vi "practica111.vi"() -> ()   [LabVIEW 2016]
panel:
  out "S2 x":dbl
  out "S2 y":dbl
  out "S1 x":dbl
  out "S1 y":dbl
  in  "S2":i32
  in  "S1":i32
  in  "stop":bool
  in  "S2":dbl(knob) scale=-175.0..175.0
  in  "S1":dbl(knob) scale=0.0..360.0
  out "XY Graph":cluster{"Y":dbl[], "Y":dbl[]}[](graph)
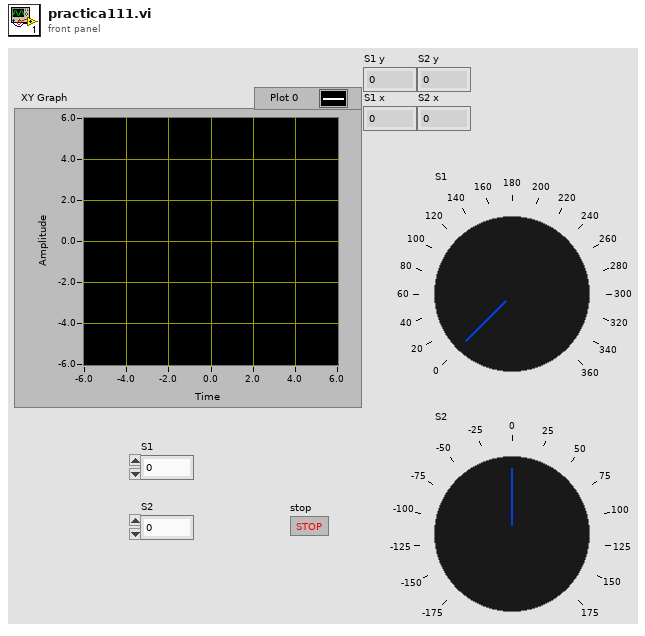
[diagram p1: front panel]
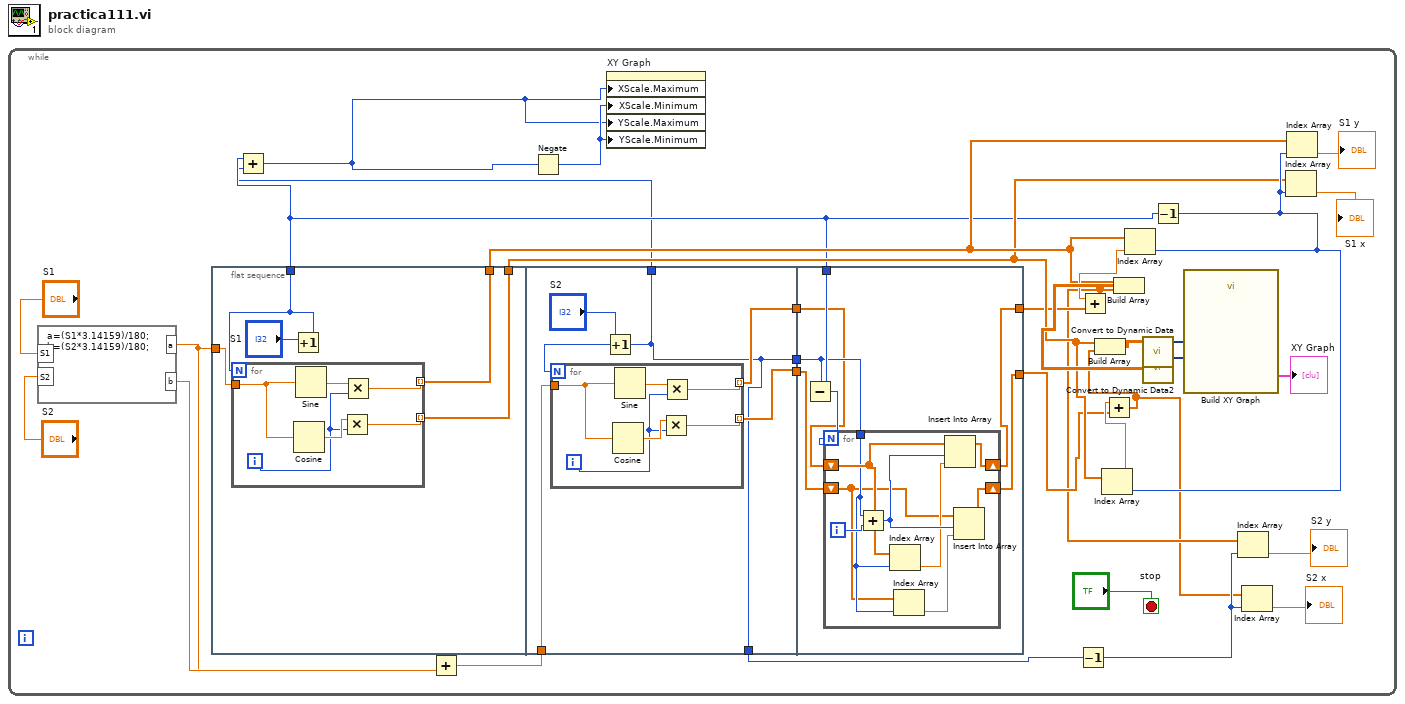
[diagram p0: block diagram]
diagram:
  n1 = while {
    stop <- "stop" stop-if-true
    n2 = formula code="a=(S1*3.14159)/180;\nb=(S2*3.14159)/180;"("S1"="S1", "S2"="S2") -> ("b"=w24:dbl, "a"=w23:dbl)
    n3 = flat-sequence {
      tunnel: w23 -> [w38]
      tunnel: [w34] -> w4
      tunnel: [w36] -> w16
      tunnel: [w35] -> w15
      tunnel: w22 -> [w48]
      tunnel: [w47] -> w20
      tunnel: [w46] -> w19
      tunnel: [w45] -> w18
      tunnel: [w45] -> w7
      tunnel: [w45] -> w3
      tunnel: [w59] -> w12
      tunnel: [w58] -> w9
      tunnel: w20 -> [w56]
      tunnel: w19 -> [w57]
      tunnel: w4 -> [w62]
      tunnel: w18 -> [w60]
      frame #0 {
        n4 = Increment(x="S1") -> (x+1=w34:i32)
        n5 = for {
          N: w34 -> [_]
          tunnel: w38 -> [w40]
          tunnel: [w42] -> w36 mode=indexing
          tunnel: [w41] -> w35 mode=indexing
          i -> [w39]
          n6 = Cosine(x=w40) -> (cos(x)=w44:dbl)
          n7 = Sine(x=w40) -> (sin(x)=w43:dbl)
          n8 = Multiply(x=w44, y=w39) -> (x*y=w41:dbl)
          n9 = Multiply(x=w43, y=w39) -> (x*y=w42:dbl)
        }
      }
      frame #1 {
        n10 = Increment(x="S2") -> (x+1=w45:i32)
        n11 = for {
          N: w45 -> [_]
          tunnel: w48 -> [w51]
          tunnel: [w53] -> w46 mode=indexing
          tunnel: [w52] -> w47 mode=indexing
          i -> [w50]
          n12 = Cosine(x=w51) -> (cos(x)=w55:dbl)
          n13 = Sine(x=w51) -> (sin(x)=w54:dbl)
          n14 = Multiply(x=w55, y=w50) -> (x*y=w52:dbl)
          n15 = Multiply(x=w54, y=w50) -> (x*y=w53:dbl)
        }
      }
      frame #2 {
        n16 = Subtract(x=w62, y=w60) -> (x-y=w61:i32)
        n17 = for {
          N: w61 -> [_]
          tunnel: w60 -> [w66]
          shift-right: [w67] -> w59
          shift-left: w57 -> [w69]
          shift-right: [w63] -> w58
          shift-left: w56 -> [w65]
          i -> [w71]
          n18 = Add(x=w66, y=w71) -> (x+y=w70:i32)
          n19 = Index Array(array=w69, index=w66) -> (element=w68:dbl)
          n20 = Index Array(array=w65, index=w66) -> (element=w64:dbl)
          n21 = Insert Into Array(array=w69, index=w70, new element=w68) -> (w67:dbl[])
          n22 = Insert Into Array(array=w65, index=w70, new element=w64) -> (w63:dbl[])
        }
      }
    }
    n23 = Add(x=w4, y=w3) -> (x+y=w1:i32)
    n24 = Add(x=w23, y=w24) -> (x+y=w22:dbl)
    n25 = Negate(x=w1) -> (-x=w2:i32)
    n26 = property on="XY Graph" class="XYGraph (strict)"("XScale.Maximum"=w1, "XScale.Minimum"=w2, "YScale.Maximum"=w1, "YScale.Minimum"=w2) -> ()  [unwired: 2 in, 2 out]
    n27 = Decrement(x=w7) -> (x-1=w8:i32)
    n28 = Decrement(x=w4) -> (x-1=w17:i32)
    n29 = Index Array(array=w15, index=w17) -> (element=w25:dbl)
    n30 = Add(x=w25, y=w9) -> (x+y=w5:dbl[])
    n31 = Build Array(w15, w5) -> (w30:dbl[][])
    n32 = Index Array(array=w16, index=w17) -> (element=w21:dbl)
    n33 = Add(x=w21, y=w12) -> (x+y=w6:dbl[])
    n34 = Build Array(w16, w6) -> (w28:dbl[][])
    n35 = call "Convert to Dynamic Data"("2D Array"=w30) -> ("Dynamic Data Type"=w29:dynamicdata)  [unwired: 3 in]
    n36 = call "Convert to Dynamic Data2"("2D Array"=w28) -> ("Dynamic Data Type"=w27:dynamicdata)  [unwired: 3 in]
    n37 = call "Build XY Graph"("Y Input"=w27, "X Input"=w29) -> ("XY Graph"=→"XY Graph":cluster{"X":dbl[], "Y":dbl[]}[])  [unwired: 8 in, 1 out]
    n38 = Index Array(array=w6, index=w8) -> (element=→"S2 y":dbl)
    n39 = Index Array(array=w5, index=w8) -> (element=→"S2 x":dbl)
    n40 = Index Array(array=w15, index=w17) -> (element=→"S1 x":dbl)
    n41 = Index Array(array=w16, index=w17) -> (element=→"S1 y":dbl)
  }
